vi "Toggle_Case.vi"(0 "Input_String":string caption="Input String", 5 "Stop":bool) -> ()   [LabVIEW 2021]
doc: "This VI Toggles the characters entered.\nIf entered char is Upper case, then convereted to Lower case.\nIf entered char is Lower case, then convereted to Uower case."
panel:
  # "TOGGLE CASE GENERATOR"
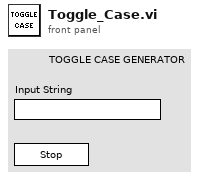
[diagram p1: front panel]
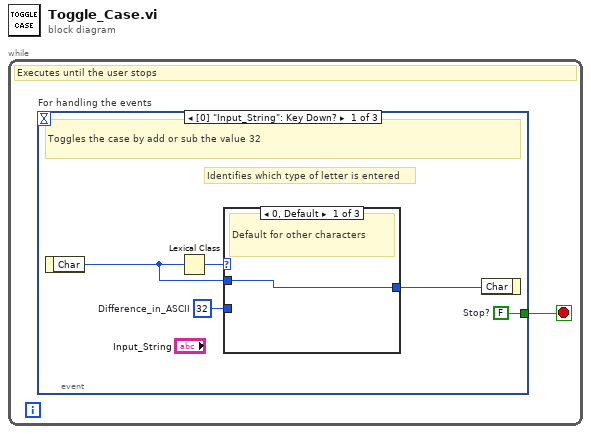
[diagram p0: block diagram]
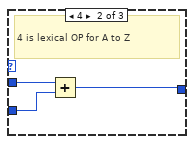
[diagram p2: hidden frame]
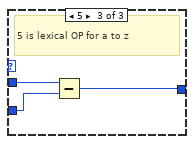
[diagram p3: hidden frame]
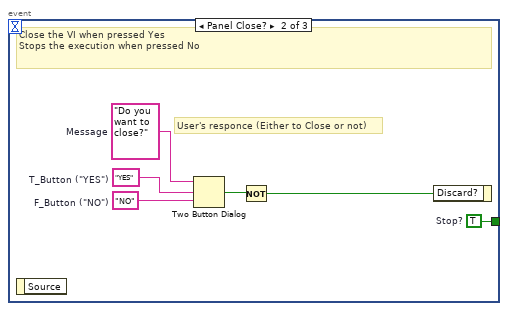
[diagram p4: hidden frame]
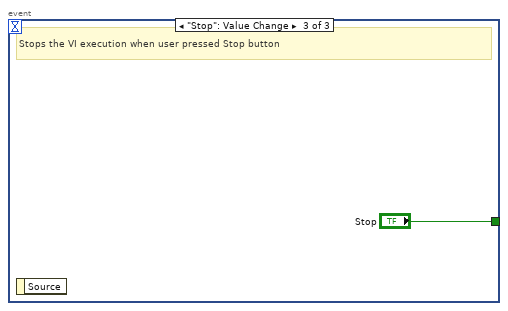
[diagram p5: hidden frame]
diagram:
  n1 = while {
    stop <- w1 stop-if-true
    # "Executes until the user stops"
    n2 = event "For handling the events" shown="[0] \"Input_String\": Key Down?" {
      selector: _ -> [_ _ _]
      dyn-events: _ -> [_ _ _]
      timeout: _ -> [_ _ _]
      tunnel: [w3 w16 "Stop"] -> w1
      event "Input_String": Key Down? {
        w3 = FALSE  # Stop?
        w4 = i16 32  # Difference_in_ASCII
        # "Identifies which type of letter is entered"
        # "Toggles the case by add or sub the value 32"
        n3 = event-data() -> ("Char"=w2:i16)  [unwired: 1 in]
        n4 = Lexical Class(1:w2) -> (0:w6:i16)
        n5 = case shown="0, Default" w6 {
          tunnel: [w7 w10 w13] -> w5
          tunnel: w2 -> [w7 w9 w12]
          tunnel: w4 -> [_ w8 w11]
          frame 0, Default {
            # "Default for other characters"
          }
          frame 4 {
            # "4 is lexical OP for A to Z"
            n6 = Add(x=w9, y=w8) -> (x+y=w10:i16)
          }
          frame 5 {
            # "5 is lexical OP for a to z"
            n7 = Subtract(x=w12, y=w11) -> (x-y=w13:i16)
          }
        }
        n8 = event-data ("Event Filter Node")("Char"=w5) -> ()  [unwired: 1 in, 1 out]
      }
      event Panel Close? {
        w14 = "NO"  # F_Button ("NO")
        w15 = "YES"  # T_Button ("YES")
        w16 = TRUE  # Stop?
        w19 = "Do you want to close?"  # Message
        # "User's responce (Either to Close or not)"
        # "Close the VI when pressed Yes\nStops the execution when pressed No"
        n9 = event-data() -> ()  [unwired: 1 in, 1 out]
        n10 = Two Button Dialog(message=w19, 1:w14, 2:w15) -> (T button?=w18:bool)
        n11 = Not(x=w18) -> (.not. x?=w17:bool)
        n12 = event-data ("Event Filter Node")("Discard?"=w17) -> ()  [unwired: 1 in, 1 out]
      }
      event "Stop": Value Change {
        # "Stops the VI execution when user pressed Stop button"
        n13 = event-data() -> ()  [unwired: 1 in, 1 out]
      }
    }
  }
